vi "ToString_ReturnsVITitle.vi"() -> ()   [LabVIEW 2019, in "FactTest.lvlib"]
uses:
  FactTest.lvlib
  Fact/Fact.lvclass
  Support/Support.lvlib
  a7e9dbe7-fcdc-4991-af27-9af2d0a95db2.vi
panel:
  out "error out":errorcluster
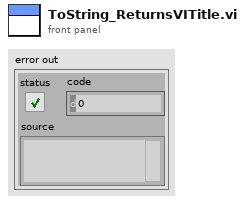
[diagram p1: front panel]
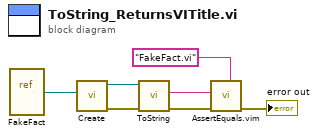
[diagram p0: block diagram]
diagram:
  n1 = vi-ref "FakeFact.vi"() -> (w3:refnum<vi>)
  n2 = call "Create.vi"("VI Refnum"=w3) -> ("error out"=w6:errorcluster, "Fact"=w7:refnum<class "Fact.lvclass">)  [unwired: 9 in]
  n3 = call-dynamic "ToString.vi"("error in (no error)"=w6, "Fact in"=w7) -> ("error out"=w5:errorcluster, "String"=w2:string)  [unwired: 7 in, 1 out]
  n4 = call "AssertEquals.vim"("Expected"="FakeFact.vi" ("String"), "error in (no error)"=w5, "Actual"=w2) -> ("error out"=→"error out":errorcluster)  [unwired: 8 in]
